vi "MCB2300G PWM ProjectAttrValidator.vi"(5 "Ctl Refnum":refnum<vi>, 7 "IO Name (original)":string, 9 "IO Channel Number":i32(ring) items=["137", "138", "139", "140", "141", "142"], 11 "Attributes":T1={"Offset%"=50, "Double edge?"=FALSE, "Polarity"=FALSE, "Programmable Pin Connections"=0, "Frequency (Hz)"=1000} {"Programmable Pin Connections" items=["PWM1 uses pin P2.0. You cannot use PWM1 and pin P2.0 in the same project.", "PWM2 uses pin P2.1. You cannot use PWM2 and pin P2.1 in the same project.", "PWM3 uses pin P2.2. You cannot use PWM3 and pin P2.2 in the same project.", "PWM4 uses pin P2.3. You cannot use PWM4 and pin P2.3 in the same project.", "PWM5 uses pin P2.4. You cannot use PWM5 and pin P2.4 in the same project.", "PWM6 uses pin P2.5. You cannot use PWM6 and pin P2.5 in the same project."]}) -> (3 "Valid?":bool)   [LabVIEW 2011]
uses:
  <vilib>/Embedded/ARM/MCB2300/MCB2300G_PWM_PrjAttr.ctl
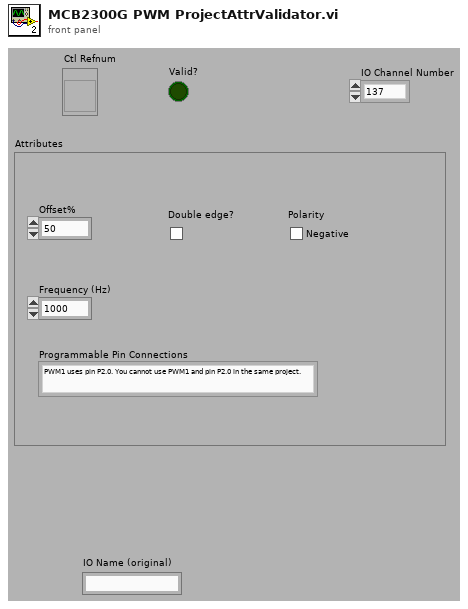
[diagram p1: front panel]
types:
  T1 = typedef "MCB2300G_PWM_PrjAttr.ctl" = cluster{"Offset%":u8, "Double edge?":bool, "Polarity":bool, "Programmable Pin Connections":u16, "Frequency (Hz)":u32}
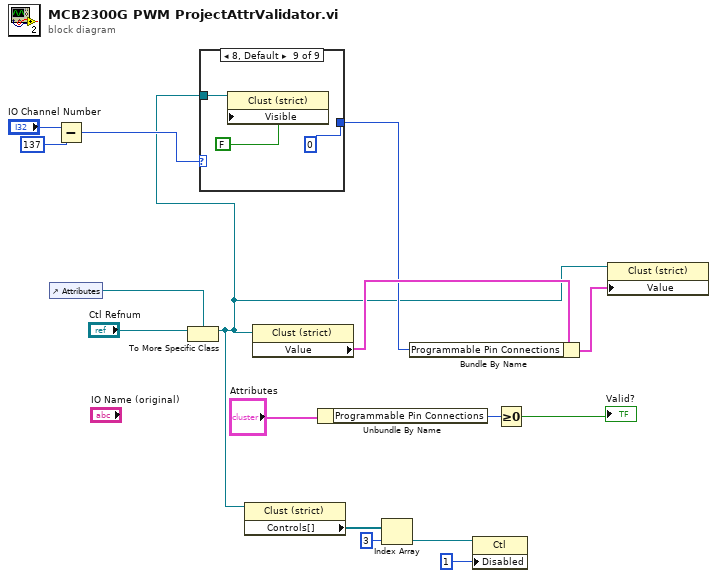
[diagram p0: block diagram]
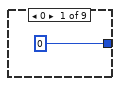
[diagram p2: hidden frame]
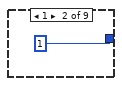
[diagram p3: hidden frame]
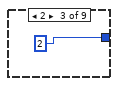
[diagram p4: hidden frame]
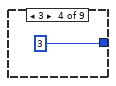
[diagram p5: hidden frame]
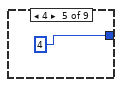
[diagram p6: hidden frame]
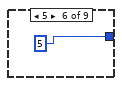
[diagram p7: hidden frame]
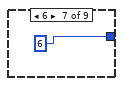
[diagram p8: hidden frame]
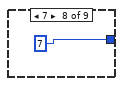
[diagram p9: hidden frame]
diagram:
  n1 = control-ref of="Attributes"() -> (w1:refnum<vi>)
  n2 = Subtract(x="IO Channel Number", y=137) -> (x-y=w5:i32)
  n3 = To More Specific Class(target class=w1, reference="Ctl Refnum") -> (specific class reference=w3:refnum<vi>)  [unwired: 1 in, 1 out]
  n4 = case shown="8, Default" w5 {
    tunnel: [0 1 2 3 4 5 6 7 0] -> w4
    tunnel: w3 -> [_ _ _ _ _ _ _ _ w25]
    frame 0 {
    }
    frame 1 {
    }
    frame 2 {
    }
    frame 3 {
    }
    frame 4 {
    }
    frame 5 {
    }
    frame 6 {
    }
    frame 7 {
    }
    frame 8, Default {
      n5 = property class="Clust (strict)"(reference=w25, "Visible"=FALSE) -> ()  [unwired: 1 in, 2 out]
    }
  }
  n6 = property class="Clust (strict)"(reference=w3) -> ("Controls[]"=w13:refnum<vi>[])  [unwired: 1 in, 2 out]
  n7 = property class="Clust (strict)"(reference=w3) -> ("Value"=w15:T1)  [unwired: 1 in, 2 out]
  n8 = Unbundle By Name("Attributes") -> ("Programmable Pin Connections"=w9:u16)
  n9 = Index Array(array=w13, index=3) -> (element=w11:refnum<vi>)
  n10 = Bundle By Name(cluster=w15, "Programmable Pin Connections"=w4) -> (w14:T1)
  n11 = property class="Ctl"(reference=w11, "Disabled"=u8 1) -> ()  [unwired: 1 in, 2 out]
  n12 = Greater Or Equal To 0?(x=w9) -> (x >= 0?=→"Valid?":bool)
  n13 = property class="Clust (strict)"(reference=w3, "Value"=w14) -> ()  [unwired: 1 in, 2 out]
